vi "FdxCmdTxQueueUpdateCvi.vi"(8 "error in":errorcluster, 9 "TxQueueUpdateIn":T1, 11 "InstrumentHandle":u32) -> (0 "error out":errorcluster, 3 "InstrumentHandle":u32)   [LabVIEW 2020, in "AIM664LV.lvlib"]
doc: "This function allows update of frames in a generic transmit queue after a frame was already written to the queue. The update is also possible while the transmission is running (on the fly). It is only possible to update AFDX- FRAME data (MAC-Frame) data and not the Fixed Header like described in AiFdxCmdTxQueueWrite."
uses:
  AIM664LV.lvlib
  AFDX_LibraryAdmin/FdxGlobalDllPath.vi
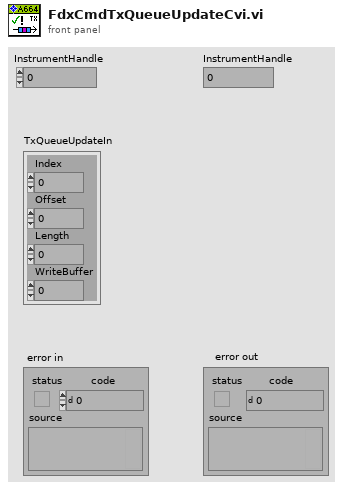
[diagram p1: front panel]
types:
  T1 = cluster{"Index":u32, "Offset":u32, "Length":u32, "WriteBuffer":u8}
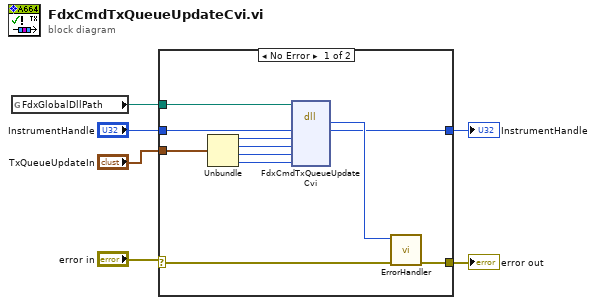
[diagram p0: block diagram]
diagram:
  n1 = global read "FdxGlobalDllPath.vi" "FdxGlobalDllPath"() -> (w4:path)
  n2 = case shown="No Error" "error in" {
    selector: "error in" -> [w16 w19]
    tunnel: [w17 w19] -> w6
    tunnel: w4 -> [w10 _]
    tunnel: "InstrumentHandle" -> [w9 w18]
    tunnel: [w8 w18] -> w2
    tunnel: "TxQueueUpdateIn" -> [w7 _]
    frame No Error {
      n3 = Unbundle(w7) -> ("Index"=w14:u32, "Offset"=w13:u32, "Length"=w12:u32, "WriteBuffer"=w11:u8)
      n4 = dll-call lib="aim_fdx.19.dll" fn="FdxCmdTxQueueUpdateCvi"(path in=w10, "InstrumentHandle"=w9, "Index"=w14, "Offset"=w13, "Length"=w12, "WriteBuffer"=w11) -> ("status"=w15:i32, "InstrumentHandle"=w8:u32)  [unwired: 5 in, 3 out]
      n5 = call "ErrorHandler.vi"("error in"=w16, "AIM Error"=w15) -> ("error out"=w17:errorcluster)  [unwired: 9 in]
    }
    frame Error {
    }
  }
  "error out" <- w6
  "InstrumentHandle" <- w2
